vi "Task Start.vi"(8 "error in (no error)":errorcluster, 11 "DataHandlerTask in":refnum<class "DataHandlerTask.lvclass">) -> (0 "error out":errorcluster, 3 "DataHandlerTask out":refnum<class "DataHandlerTask.lvclass">)   [LabVIEW 2020, in "VolatusData.lvlib" / "DataHandlerTask.lvclass"]
uses:
  DataHandlerTask.lvclass
  DataHandlerTask.lvclass/DataHandlerTask.ctl
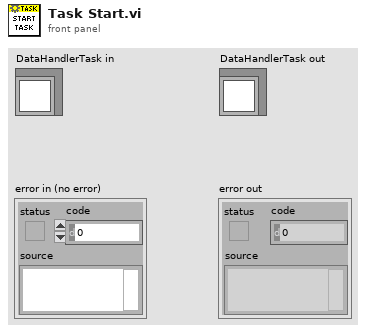
[diagram p1: front panel]
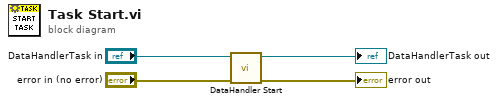
[diagram p0: block diagram]
diagram:
  n1 = call-dynamic "DataHandler Start.vi"("error in (no error)"="error in (no error)", "DataHandlerTask in"="DataHandlerTask in") -> ("error out"=→"error out":errorcluster, "DataHandlerTask out"=→"DataHandlerTask out":refnum<class "DataHandlerTask.lvclass">)  [unwired: 8 in]
